vi "Send 1_CreateClient.vi"(7 "Priority":T2=enum."Normal" caption="Message Priority (Normal)", 8 "error in (no error)":errorcluster, 10 "Create":T1={"address"="localhost", "port"=1883, "UserName"="", "Pwd"=""}, 11 "Message Enqueuer in":refnum<class "Message Enqueuer.lvclass">) -> (0 "error out":errorcluster, 3 "Message Enqueuer out":refnum<class "Message Enqueuer.lvclass">)   [LabVIEW 2018, in "MQTT_Client_Actor.lvlib" / "1_CreateClient Msg.lvclass"]
doc: "Sends the <b>MQTT_Client_Actor.lvlib:1_CreateClient Msg.lvclass</b> message.\n\nThis message will call <b>1_CreateClient.vi</b> on the <b>MQTT_Client_Actor.lvlib:MQTT_Client_Actor.lvclass</b> actor.\n\n<b>1_CreateClient.vi Description</b>"
uses:
  1_CreateClient Msg.lvclass
  <vilib>/ActorFramework/Message Enqueuer/Message Enqueuer.lvclass
  <vilib>/ActorFramework/Message Enqueuer/Message Priority.ctl
  MQTT_Client_Actor/CreateClient.ctl
  D:/Program Files (x86)/National Instruments/LabVIEW 2018/vi.lib/ActorFramework/Message/Message.lvclass
  1_CreateClient Msg.lvclass/1_CreateClient Msg.ctl
  <vilib>/ActorFramework/Message Enqueuer/Message Enqueuer.lvclass/Message Enqueuer.ctl
  <vilib>/ActorFramework/Message Priority Queue/Priority Enqueue.vi
  MQTT_Client_Actor/MQTT_Client_Actor.lvclass
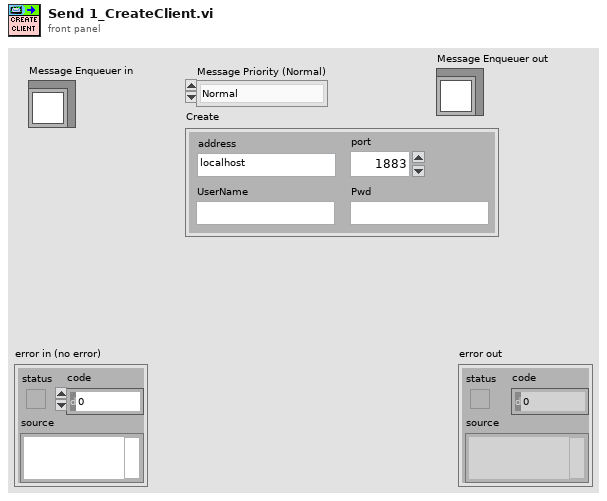
[diagram p1: front panel]
types:
  T1 = typedef "MQTT_Client_Actor.lvlib/MQTT_Client_Actor.lvclass/CreateClient.ctl" = cluster{"address":string, "port":u16, "UserName":string, "Pwd":string}
  T2 = typedef "Actor Framework.lvlib/Message Enqueuer.lvclass/Message Priority.ctl" = enum16{"Low", "Normal", "High"}
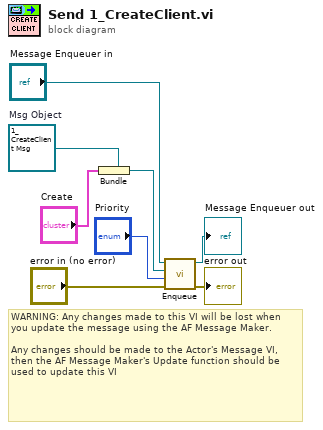
[diagram p0: block diagram]
diagram:
  w7 = refnum<class "1_CreateClient Msg.lvclass"> refnum  # Msg Object
  # "WARNING: Any changes made to this VI will be lost when you update the message using the AF Message Maker.\n\nAny changes should be made to the Actor's Message VI, then the AF Message Maker's Update function should be used to update this VI"
  n1 = Bundle(cluster=w7, "Create") -> (w2:refnum<class "1_CreateClient Msg.lvclass">)
  n2 = call <vilib>:"Enqueue.vi"("error in (no error)"="error in (no error)", "Message Priority (Normal)"="Priority", "Message"=w2, "Message Enqueuer in"="Message Enqueuer in") -> ("error out"=→"error out":errorcluster, "Message Enqueuer out"=→"Message Enqueuer out":refnum<class "Message Enqueuer.lvclass">)  [unwired: 6 in]
